vi "Initialize.vi"(8 "error in":errorcluster, 10 "resource":string, 11 "host in":refnum<class "LIA Host Interface FPGA.lvclass">) -> (0 "error out":errorcluster, 3 "host out":refnum<class "LIA Host Interface FPGA.lvclass">)   [LabVIEW 2018, in "LIA Host Interface FPGA.lvclass"]
uses:
  LIA Host Interface FPGA.lvclass
  Session Data.ctl
  LIA Host Interface FPGA.lvclass/LIA Host Interface FPGA.ctl
  <vilib>/FPGAPlugInAG/PXIe-7976R/niLvFpga_Open_PXIe-7976R.vi
  <vilib>/rvi/interface/common/dynamic/niFpgaDynamicAddResources.vi
  <vilib>/FPGAPlugInAG/NI-7935R/niLvFpga_Open_NI-7935R.vi
  <vilib>/Utility/error.llb/Error Cluster From Error Code.vi
  <vilib>/rvi/errors/niLvFpgaAdjustHostInterfaceError.vi
  <vilib>/rvi/interface/nirviOpenFPGA/nirviOpenFPGA.xnode
  targets/7976/bitfiles/LIA 7976 5783.lvbitx
  targets/7935/bitfiles/LIA 7935 5783.lvbitx
  <vilib>/rvi/interface/nirviReadWriteControl/nirviReadWriteControl.xnode
  host/Lock-In Amplifier Example Host.lvlib
  NiFpgaLv.dll
  <vilib>/rvi/interface/Simulation/niFpgaSimulationCallBeginRW.vi
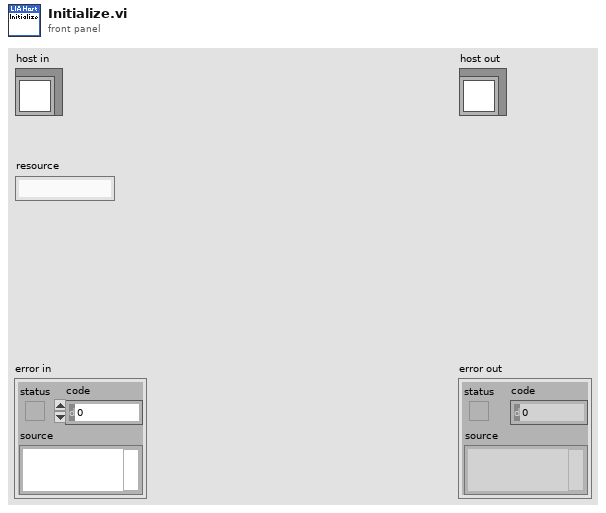
[diagram p1: front panel]
types:
  T1 = typedef "LIA Host Interface FPGA.lvclass/Session Data.ctl" = cluster{"fpga session":refnum<k20>, "record length":u32[]}
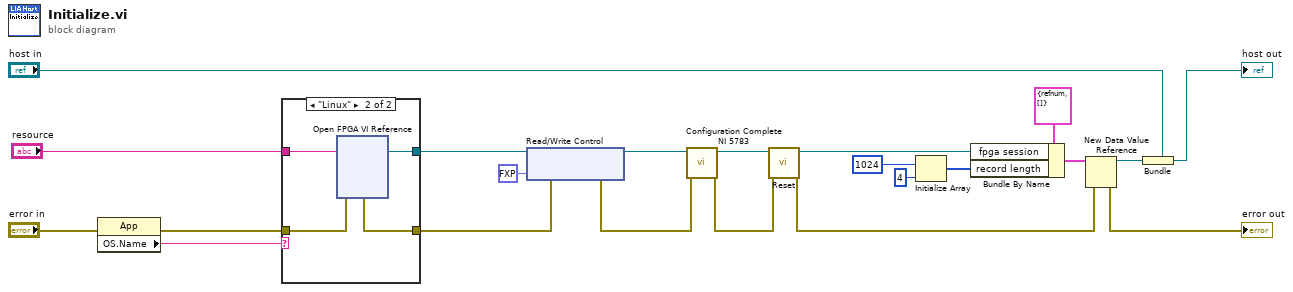
[diagram p0: block diagram]
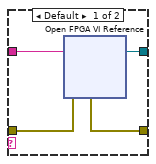
[diagram p2: hidden frame]
diagram:
  n1 = property class="App"(error in="error in") -> (error out=w2:errorcluster, "OS.Name"=w1:string)  [unwired: 1 in, 1 out]
  n2 = case shown="\"Linux\"" w1 {
    tunnel: "resource" -> [w25 w30]
    tunnel: [w26 w29] -> w13
    tunnel: [w23 w28] -> w9
    tunnel: w2 -> [w24 w27]
    frame Default {
      n3 = xnode "Open FPGA VI Reference"("error in"=w24, "resource name"=w25) -> ("FPGA VI Reference Out"=w26:refnum<k20>, "error out"=w23:errorcluster)
    }
    frame "Linux" {
      n4 = xnode "Open FPGA VI Reference"("error in"=w27, "resource name"=w30) -> ("FPGA VI Reference Out"=w29:refnum<k20>, "error out"=w28:errorcluster)
    }
  }
  n5 = xnode "Read/Write Control"("FPGA VI Reference In"=w13, "error in"=w9, "ao.noise gain 3"=fxp<+,18,1> 0.0) -> ("FPGA VI Reference Out"=w10:refnum<k20>, "error out"=w8:errorcluster)
  n6 = call "Configuration Complete NI 5783.vi"("error in"=w8, "fpga session in"=w10) -> ("error out"=w12:errorcluster, "fpga session out"=w11:refnum<k20>)  [unwired: 7 in, 1 out]
  n7 = call "Reset.vi"("error in"=w12, "fpga session in"=w11) -> ("error out"=w18:errorcluster, "fpga session out"=w21:refnum<k20>)  [unwired: 8 in]
  n8 = Initialize Array(u32 1024 ("element"), 4 ("dimension size")) -> (w4:u32[])
  n9 = Bundle By Name(cluster=T1 {"fpga session"=refnum, "record length"=[]} ("session data"), "fpga session"=w21, "record length"=w4) -> (w19:T1)
  n10 = New Data Value Reference(data value=w19, error in=w18) -> (data value reference=w16:refnum<data-value>, error out=→"error out":errorcluster)
  n11 = Bundle(cluster="host in", w16) -> (→"host out":refnum<class "LIA Host Interface FPGA.lvclass">)
